vi "Imports.vi"(6 "error in":errorcluster, 9 "PythonConverter_GUI in":refnum<class "PythonConverter_GUI.lvclass">) -> (0 "error out":errorcluster, 3 "PythonConverter_GUI out":refnum<class "PythonConverter_GUI.lvclass">, 4 "imports":string)   [LabVIEW 2014, in "PythonConverter_GUI.lvclass"]
uses:
  PythonConverter_GUI.lvclass
  PythonConverter_GUI.lvclass/PythonConverter_GUI.ctl
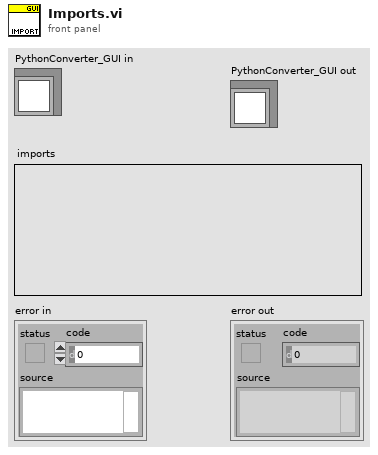
[diagram p1: front panel]
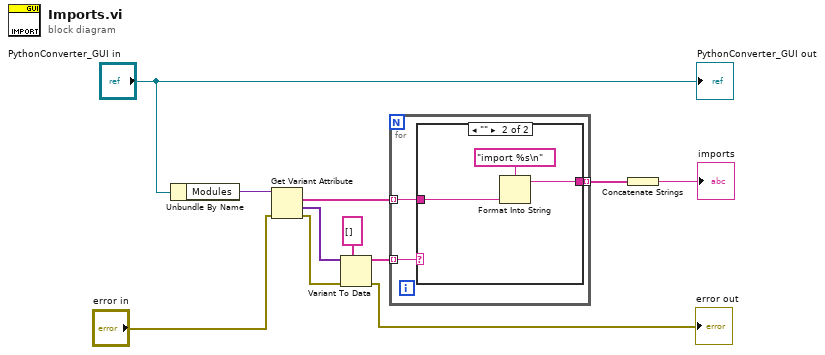
[diagram p0: block diagram]
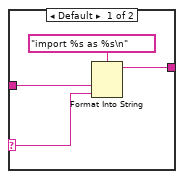
[diagram p2: hidden frame]
diagram:
  n1 = Unbundle By Name("PythonConverter_GUI in") -> ("Modules"=w11:variant)
  n2 = Get Variant Attribute(Variant=w11, error in="error in") -> (names=w7:string[], values=w10:variant[], error out=w5:errorcluster)  [unwired: 2 in, 1 out]
  n3 = Variant To Data(error in=w5, type=string[] [], Variant=w10) -> (data=w8:string[], error out=→"error out":errorcluster)
  n4 = for {
    tunnel: w8 -> [w12] mode=indexing
    tunnel: w7 -> [w14] mode=indexing
    tunnel: [w13] -> w6 mode=indexing
    n5 = case shown="\"\"" w12 {
      selector: w12 -> [w15 _]
      tunnel: w14 -> [w18 w21]
      tunnel: [w16 w19] -> w13
      frame Default {
        n6 = Format Into String(format string="import %s as %s\n", w18, w15) -> (resulting string=w16:string)  [unwired: 2 in, 1 out]
      }
      frame "" {
        n7 = Format Into String(format string="import %s\n", w21) -> (resulting string=w19:string)  [unwired: 2 in, 1 out]
      }
    }
  }
  n8 = Concatenate Strings(w6) -> (→"imports":string)
  "PythonConverter_GUI out" <- "PythonConverter_GUI in"
